vi "GenFolder.vi"(2 "error in (no error)":errorcluster, 3 "name or relative path":string) -> (0 "error out":errorcluster, 1 "dup path":path)   [LabVIEW 2012, in "EpiWrapper.lvclass"]
uses:
  EpiWrapper.lvclass
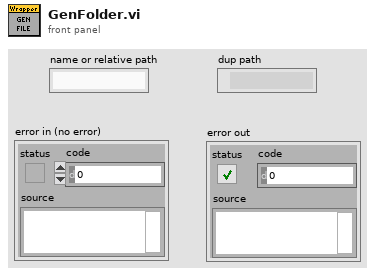
[diagram p1: front panel]
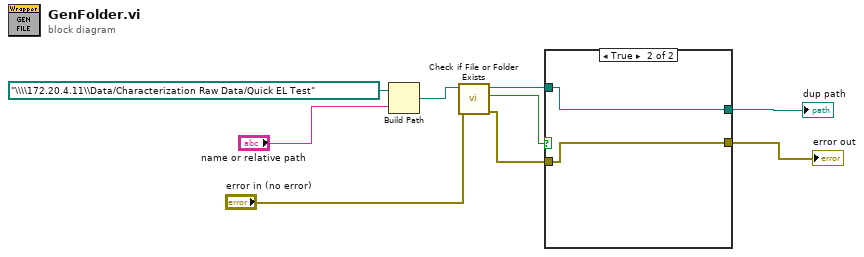
[diagram p0: block diagram]
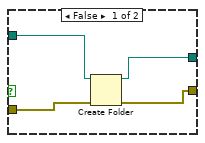
[diagram p2: hidden frame]
diagram:
  n1 = Build Path(base path=path "\\\\172.20.4.11\\Data/Characterization Raw Data/Quick EL Test", name or relative path="name or relative path") -> (appended path=w7:path)
  n2 = call <vilib>:"Check if File or Folder Exists.vi"("error in (no error)"="error in (no error)", "path"=w7) -> ("error out"=w4:errorcluster, "file or folder exists?"=w6:bool, "dup path"=w5:path)  [unwired: 7 in]
  n3 = case shown="True" w6 {
    tunnel: w5 -> [w13 w15]
    tunnel: w4 -> [w12 w14]
    tunnel: [w11 w15] -> w3
    tunnel: [w10 w14] -> w2
    frame False {
      n4 = Create Folder(path (use dialog)=w13, error in=w12) -> (created path=w11:path, error out=w10:errorcluster)  [unwired: 1 in, 1 out]
    }
    frame True {
    }
  }
  "dup path" <- w3
  "error out" <- w2
